vi "Parametric graph.vi"() -> ()   [LabVIEW 2016]
uses:
  <vilib>/Analysis/6fits.llb/Prediction Interval (Gauss).vi
  <vilib>/Analysis/NI_AALPro.lvlib
panel:
  out "Boolean":bool
  in  "TestStand UI SequenceView Control":refnum<k7>(container)
  in  "stop":bool
  out "Observed Data and Fitted Curve":cluster{cluster{dbl, "Numeric":dbl}[]}[](graph)
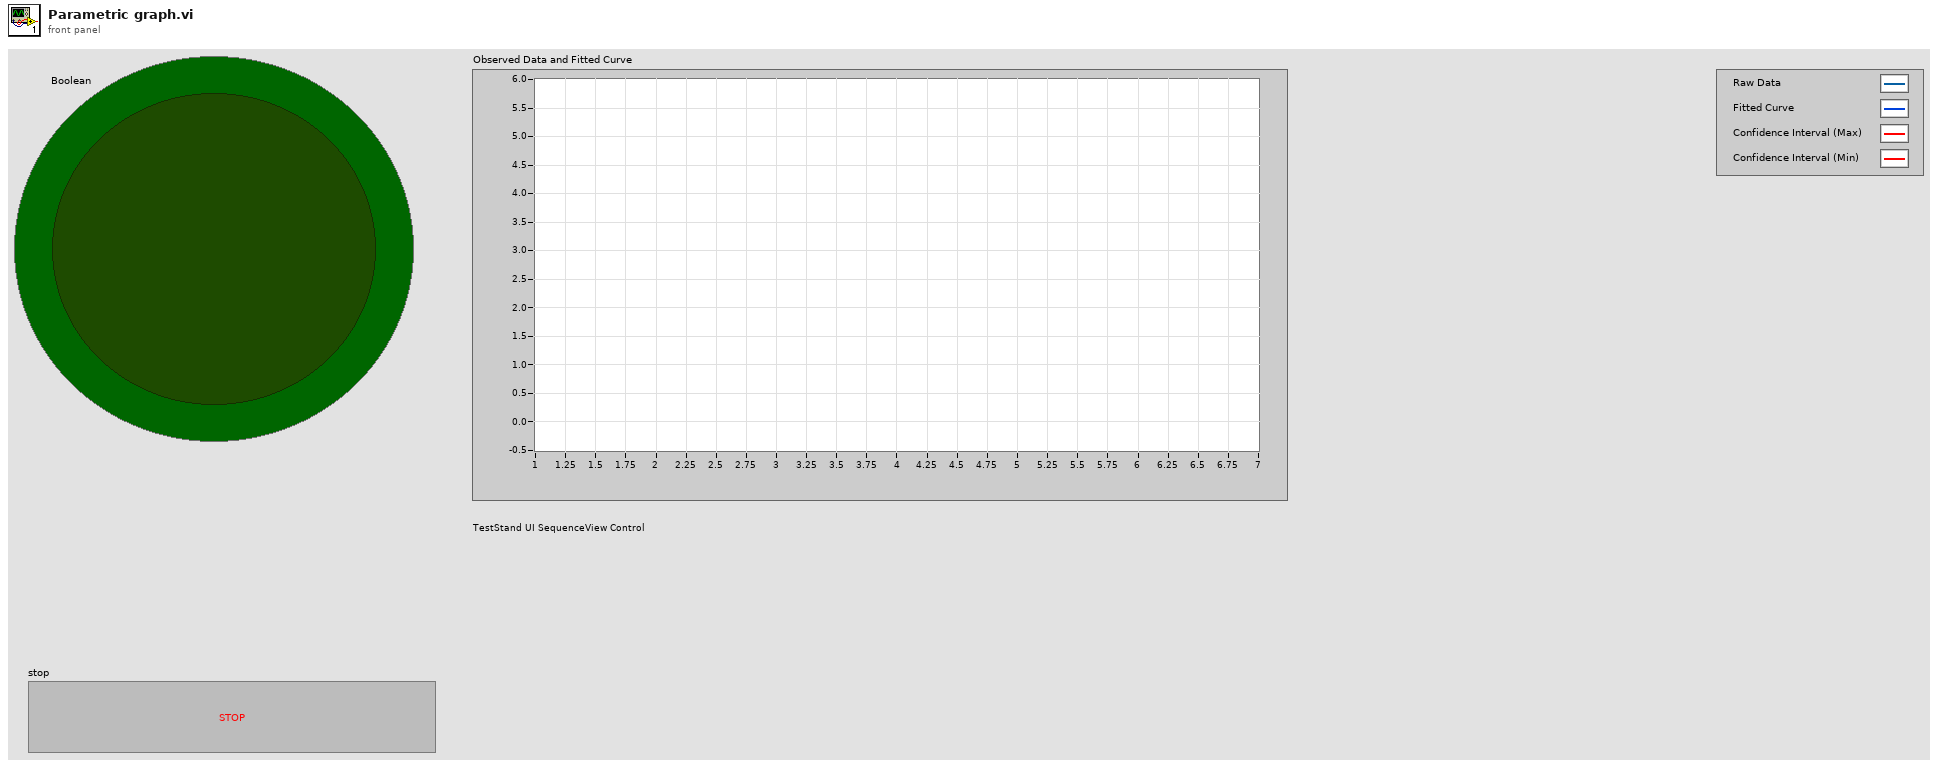
[diagram p1: front panel]
types:
  T1 = enum16{"Linear", "Exponential", "Power", "Gaussian", "Logarithmic"}
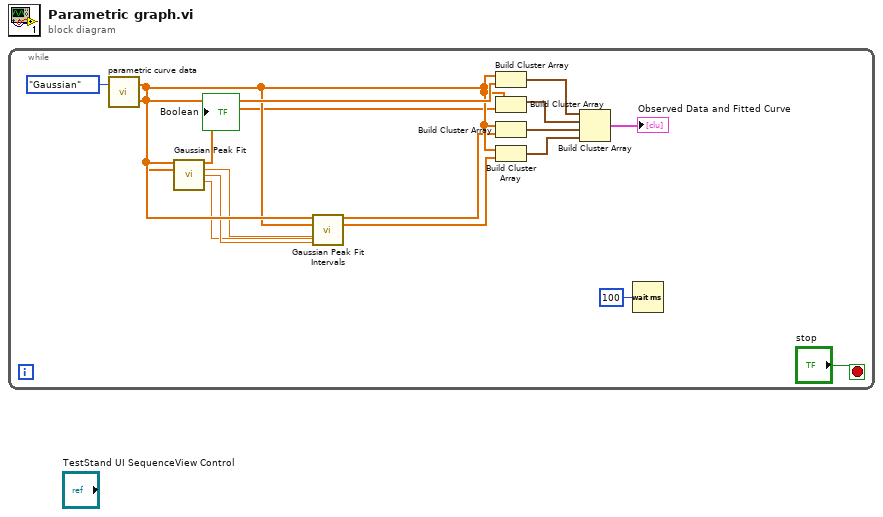
[diagram p0: block diagram]
diagram:
  n1 = while {
    stop <- "stop" stop-if-true
    n2 = call "parametric curve data.vi"("Signal type"=T1."Gaussian") -> ("Y"=w10:dbl[], "X"=w9:dbl[])  [unwired: 1 in]
    n3 = call <vilib>:"Gaussian Peak Fit.vi"("Y"=w10, "X"=w9) -> ("Best Gaussian Fit"=w8:dbl[], "amplitude"=w5:dbl, "center"=w4:dbl, "standard deviation"=w3:dbl)  [unwired: 7 in, 3 out]
    n4 = call-poly <vilib>:"Gaussian Peak Fit Intervals.vi"("Y"=w10, "X"=w9, "amplitude"=w5, "center"=w4, "standard deviation"=w3) -> ("Upper Bound"=w7:dbl[], "Lower Bound"=w6:dbl[])  [unwired: 8 in, 1 out]
    n5 = Build Cluster Array(w9, w10) -> (w13:cluster{dbl, dbl}[])
    n6 = Build Cluster Array(w9, w8) -> (w12:cluster{dbl, "Numeric":dbl}[])
    n7 = Build Cluster Array(w9, w7) -> (w15:cluster{dbl, "Numeric":dbl}[])
    n8 = Build Cluster Array(w9, w6) -> (w14:cluster{dbl, "Numeric":dbl}[])
    n9 = Build Cluster Array(w13, w12, w15, w14) -> (→"Observed Data and Fitted Curve":cluster{cluster{dbl, "Numeric":dbl}[]}[])
    n10 = Wait (ms)(milliseconds to wait=u32 100) -> ()  [unwired: 1 out]
  }
